vi "CompVisionUtil_EstimateCameraToTarget.vi"(9 "GyroAngle":T1={"VALUE"=0.0, "COS"=1.0, "SIN"=0.0} {"SIN" format="%13.4f"; "COS" format="%13.4f"; "VALUE" format="%13.4f"}, 10 "FieldToTarget":T4={"TRANSLATION"={"X"=0.0, "Y"=0.0}, "ROTATION"={"VALUE"=0.0, "COS"=1.0, "SIN"=0.0}} {"ROTATION"."SIN" format="%13.4f"; "ROTATION"."COS" format="%13.4f"; "ROTATION"."VALUE" format="%13.4f"; "TRANSLATION"."Y" format="%14.3f"; "TRANSLATION"."X" format="%14.3f"}, 11 "CameraToTargetTranslation":T3 {"Y" format="%14.3f"; "X" format="%14.3f"}) -> (3 "EstimateCameraToTarget":T2={"TRANSLATION"={"X"=0.0, "Y"=0.0}, "ROTATION"={"VALUE"=0.0, "COS"=1.0, "SIN"=0.0}} {"ROTATION"."SIN" format="%13.4f"; "ROTATION"."COS" format="%13.4f"; "ROTATION"."VALUE" format="%13.4f"; "TRANSLATION"."Y" format="%14.3f"; "TRANSLATION"."X" format="%14.3f"})   [LabVIEW 2019, in "Trajectory_Library.lvlib"]
doc: "Estimates a Transform2d that maps the camera position to the target position, using the robot's gyro. Note that the gyro angle provided *must* line up with the field coordinate system -- that is, it should read zero degrees when pointed towards the opposing alliance station, and increase as the robot rotates CCW.\n \nInputs: \n - CameraToTargetTranslation -- A Translation2d that encodes the x/y position \n of the target relative to the camera.\n - FieldToTarget -- A Pose2d representing the target position in the field coordinate \n system.\n - GyroAngle -- The current robot gyro angle, likely from odometry.\n\nOutputs:\n - EstimateCameraToTarget -- A Transform2d that takes us from the camera to \n the target."
uses:
  Trajectory_Library.lvlib
  TRANSLATION2D.ctl
  ROTATION2D.ctl
  POSE2D.ctl
  TRANSFORM2D.ctl
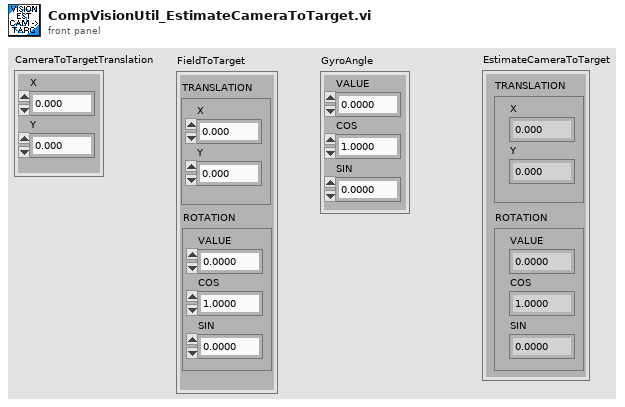
[diagram p1: front panel]
types:
  T1 = typedef "Trajectory_Library.lvlib/ROTATION2D.ctl" = cluster{"VALUE":dbl, "COS":dbl, "SIN":dbl}
  T2 = typedef "Trajectory_Library.lvlib/TRANSFORM2D.ctl" = cluster{"TRANSLATION":T3, "ROTATION":T1}
  T3 = typedef "Trajectory_Library.lvlib/TRANSLATION2D.ctl" = cluster{"X":dbl, "Y":dbl}
  T4 = typedef "Trajectory_Library.lvlib/POSE2D.ctl" = cluster{"TRANSLATION":T3, "ROTATION":T1}
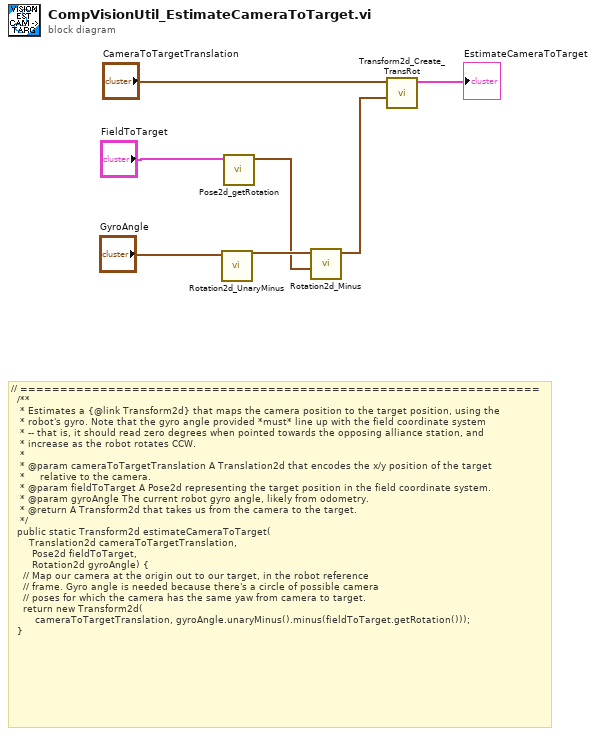
[diagram p0: block diagram]
diagram:
  # "// =================================================================\n  /**\n   * Estimates a {@link Transform2d} that maps the camera position to the target position, using the\n   * robot's gyro. Note that the gyro angle provided *must* line up with the field coordinate system\n   * -- that is, it should read zero degrees when pointed towards the opposing alliance station, and\n   * increase as the robot rotates CCW.\n   *\n   * @param cameraToTargetTranslation A Translation2d that encodes the x/y position of the target\n   *     relative to the camera.\n   * @param fieldToTarget A Pose2d representing the target position in the field coordinate system.\n   * @param gyroAngle The current robot gyro angle, likely from odometry.\n   * @return A Transform2d that takes us from the camera to the target.\n   */\n  public static Transform2d estimateCameraToTarget(\n      Translation2d cameraToTargetTranslation, \n       Pose2d fieldToTarget, \n       Rotation2d gyroAngle) {\n    // Map our camera at the origin out to our target, in the robot reference\n    // frame. Gyro angle is needed because there's a circle of possible camera\n    // poses for which the camera has the same yaw from camera to target.\n    return new Transform2d(\n        cameraToTargetTranslation, gyroAngle.unaryMinus().minus(fieldToTarget.getRotation()));\n  }"
  n1 = call "Rotation2d_UnaryMinus.vi"("in ROTATION"="GyroAngle") -> ("out ROTATION"=w4:T1)  [unwired: 10 in]
  n2 = call "Pose2d_getRotation.vi"("in POSE"="FieldToTarget") -> ("out ROTATION"=w2:T1)  [unwired: 10 in]
  n3 = call "Rotation2d_Minus.vi"("other ROTATION"=w2, "in ROTATION"=w4) -> ("out ROTATION"=w1:T1)  [unwired: 9 in]
  n4 = call "Transform2d_Create_TransRot.vi"("ROTATION"=w1, "TRANSLATION"="CameraToTargetTranslation") -> ("TRANSFORM"=→"EstimateCameraToTarget":T2)  [unwired: 9 in]
